vi "Get Rx UDP All Channels.vi"(8 "error in":errorcluster, 11 "custom device ref in":T1 format="%.0x") -> (0 "error out":errorcluster, 2 "Rx UDP channel refs":T1[](array[typedef]) format="%.0x", 3 "custom device ref out":T1 format="%.0x")   [LabVIEW 2020, in "AIM ARINC 664 Scripting.lvlib"]
uses:
  AIM ARINC 664 Scripting.lvlib
  <vilib>/NI VeriStand/Custom Device API/Custom Device Item Ref.ctl
  Constants.vi
  <vilib>/NI VeriStand/Custom Device Tools/Custom Device Utility Library/NI VeriStand - Search for All Items by GUID.vi
  <vilib>/NI VeriStand/Custom Device Tools/Custom Device Utility Library/NI VeriStand - Search for Item by GUID.vi
  <vilib>/NI VeriStand/Custom Device Tools/Custom Device Utility Library/Custom Device Utility Library.lvlib
  <vilib>/NI VeriStand/Custom Device API/Custom Device API.lvlib
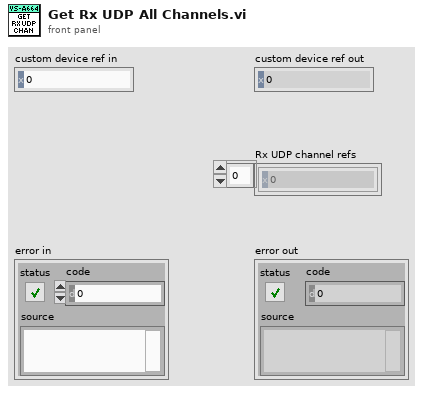
[diagram p1: front panel]
types:
  T1 = typedef "Custom Device API.lvlib/Custom Device Item Ref.ctl" = u64
  T2 = typedef "Custom Device API.lvlib/Custom Device Item Info.ctl" = cluster{"Name":string, "Is Channel":bool, "GUID":string, "Is Waveform":bool}
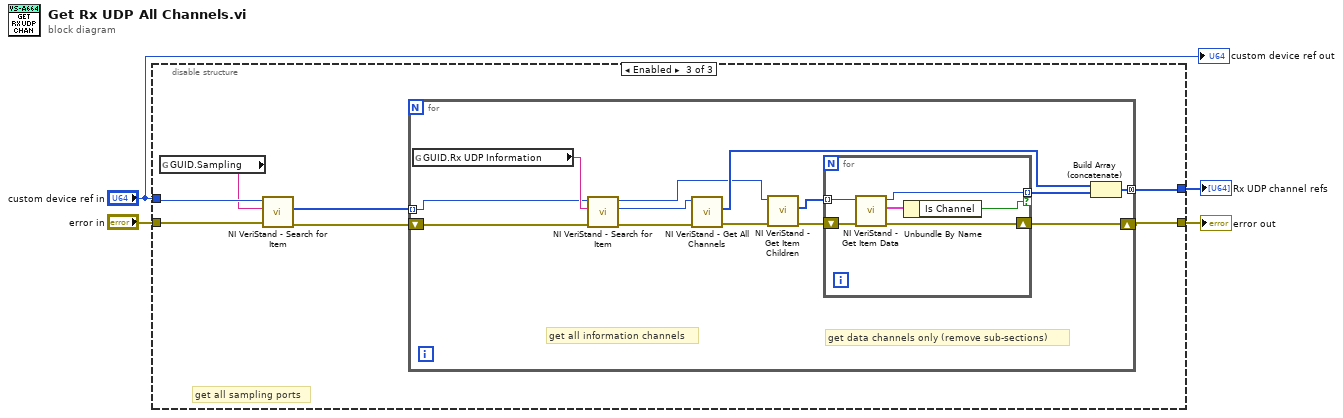
[diagram p0: block diagram]
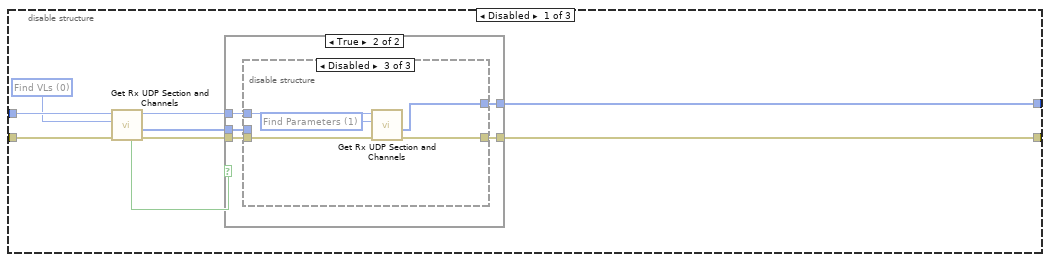
[diagram p2: hidden frame]
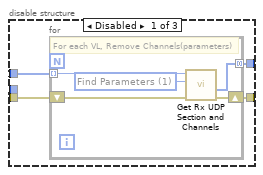
[diagram p4: hidden frame]
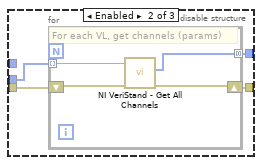
[diagram p5: hidden frame]
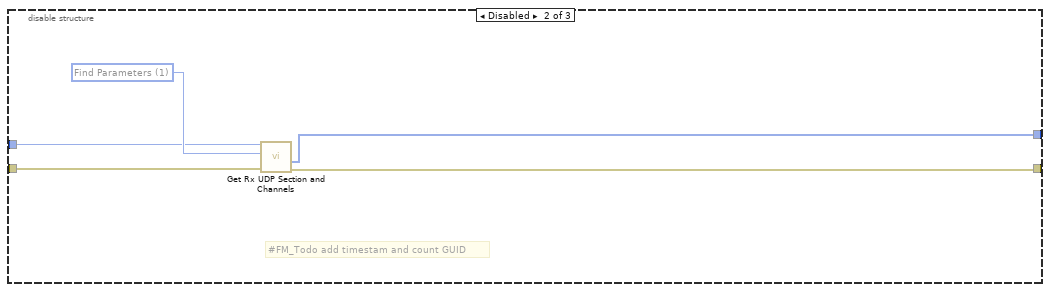
[diagram p6: hidden frame]
diagram:
  n1 = disable-structure shown="Enabled" {
    disable-tunnel: [w13 w43 w47] -> w4
    disable-tunnel: [w11 w42 w48] -> w3
    disable-tunnel: "error in" -> [w9 w44 w52]
    disable-tunnel: "custom device ref in" -> [w8 w45 w53]
    frame Disabled {
      w6 = u16 0 items=["Find VLs", "Find Parameters"] ("Option")
      n2 = call "Get Rx UDP Section and Channels.vi"("error in"=w9, "option"=w6, "custom device ref in"=w8) -> ("error out"=w12:errorcluster, "Rx UDP channel refs"=w10:T1[], "custom device ref out"=w7:T1, "found?"=w5:bool)  [unwired: 4 in, 1 out]
      n3 = case shown="True" w5 {
        tunnel: [w14 w19] -> w13
        tunnel: w12 -> [w14 w18]
        tunnel: [_ w17] -> w11
        tunnel: w10 -> [_ w16]
        tunnel: w7 -> [_ w15]
        frame False {
        }
        frame True {
          n4 = disable-structure shown="Disabled" {
            disable-tunnel: [w23 w32 w40] -> w19
            disable-tunnel: w18 -> [w22 w31 w41]
            disable-tunnel: [w21 w30 w38] -> w17
            disable-tunnel: w16 -> [w20 w29 _]
            disable-tunnel: w15 -> [_ _ w39]
            frame Disabled {
              n5 = for {
                tunnel: w20 -> [w28] mode=indexing
                tunnel: [w26] -> w21 mode=concatenating
                shift-right: [w24] -> w23
                shift-left: w22 -> [w25]
                w27 = u16 1 items=["Find VLs", "Find Parameters"] ("Option")
                # "For each VL, Remove Channels(parameters)"
                n6 = call "Get Rx UDP Section and Channels.vi"("error in"=w25, "option"=w27, "custom device ref in"=w28) -> ("error out"=w24:errorcluster, "Rx UDP channel refs"=w26:T1[])  [unwired: 4 in, 3 out]
              }
            }
            frame Enabled {
              n7 = for {
                tunnel: w29 -> [w35] mode=indexing
                tunnel: [w33] -> w30 mode=concatenating
                shift-right: [w34] -> w32
                shift-left: w31 -> [w36]
                # "For each VL, get channels (params)"
                n8 = call <vilib>:"NI VeriStand - Get All Channels.vi"("error in"=w36, "Section Ref in"=w35) -> ("error out"=w34:errorcluster, "Channel Refs"=w33:T1[])  [unwired: 6 in, 2 out]
              }
            }
            frame Disabled {
              w37 = u16 1 items=["Find VLs", "Find Parameters"] ("Option")
              n9 = call "Get Rx UDP Section and Channels.vi"("error in"=w41, "option"=w37, "custom device ref in"=w39) -> ("error out"=w40:errorcluster, "Rx UDP channel refs"=w38:T1[])  [unwired: 4 in, 3 out]
            }
          }
        }
      }
    }
    frame Disabled {
      w46 = u16 1 items=["Find VLs", "Find Parameters"] ("Option")
      # "#FM_Todo add timestam and count GUID"
      n10 = call "Get Rx UDP Section and Channels.vi"("error in"=w44, "option"=w46, "custom device ref in"=w45) -> ("error out"=w43:errorcluster, "Rx UDP channel refs"=w42:T1[])  [unwired: 4 in, 3 out]
    }
    frame Enabled {
      # "get all sampling ports"
      n11 = global read "Constants.vi" "GUID.Sampling"() -> (w51:string)
      n12 = call-poly <vilib>:"NI VeriStand - Search for Item.vi"("error in"=w52, "Item GUID"=w51, "Section Ref in"=w53) -> ("error out"=w49:errorcluster, "Item Refs"=w50:T1[])  [unwired: 5 in, 2 out]
      n13 = for {
        tunnel: w50 -> [w58] mode=indexing
        shift-right: [w59] -> w47
        shift-left: w49 -> [w66]
        tunnel: [w55] -> w48 mode=concatenating
        # "get data channels only (remove sub-sections)"
        # "get all information channels"
        n14 = global read "Constants.vi" "GUID.Rx UDP Information"() -> (w65:string)
        n15 = call-poly <vilib>:"NI VeriStand - Search for Item.vi"("error in"=w66, "Item GUID"=w65, "Section Ref in"=w58) -> ("error out"=w64:errorcluster, "Item Ref"=w63:T1, "Section Ref out"=w54:T1)  [unwired: 5 in, 1 out]
        n16 = call <vilib>:"NI VeriStand - Get All Channels.vi"("error in"=w64, "Section Ref in"=w63) -> ("error out"=w62:errorcluster, "Channel Refs"=w57:T1[])  [unwired: 6 in, 2 out]
        n17 = call <vilib>:"NI VeriStand - Get Item Children.vi"("error in (no error)"=w62, "Item Ref in"=w54) -> ("error out"=w61:errorcluster, "Child Refs"=w60:T1[])  [unwired: 6 in, 2 out]
        n18 = for {
          shift-right: [w67] -> w59
          shift-left: w61 -> [w68]
          tunnel: w60 -> [w72] mode=indexing
          tunnel: [w70] -> w56 mode=indexing if=w69
          n19 = call <vilib>:"NI VeriStand - Get Item Data.vi"("error in (no error)"=w68, "Item Ref in"=w72) -> ("error out"=w67:errorcluster, "Item Info"=w71:T2, "Item Ref out"=w70:T1)  [unwired: 7 out]
          n20 = Unbundle By Name(w71) -> ("Is Channel"=w69:bool)
        }
        n21 = Build Array (concatenate)(w57, w56) -> (w55:T1[])
      }
    }
  }
  "error out" <- w4
  "Rx UDP channel refs" <- w3
  "custom device ref out" <- "custom device ref in"
